vi "LVClass_HasoSlopes ctor from copy.vi"(0 "HasoSlopes in":refnum<class "HasoSlopes.lvclass">, 5 "HasoSlopes copy":refnum<class "HasoSlopes.lvclass">, 11 "error in (no error)":errorcluster) -> (4 "HasoSlopes out":refnum<class "HasoSlopes.lvclass">, 15 "error out":errorcluster)   [LabVIEW 2020, in "HasoSlopes.lvclass"]
doc: "HasoSlopes constructor from copy.\n\n--------------------------------------------------------------------------------\n\n<B>HasoSlopesIn </B> : Constant Pointer to HasoSlopes object.\n<B>HasoSlopesOut </B> : Constant Pointer to HasoSlopes object.\n<B>HasoSlopes_src </B> : Pointer to HasoSlopes object to copy.\n<B>ErrorIn </B> : Error\n<B>ErrorOut </B> : Error\n\n--------------------------------------------------------------------------------"
uses:
  HasoSlopes.lvclass
  Handle creation.ctl
  HasoSlopes.lvclass/HasoSlopes.ctl
  LVClass_HasoSlopes Read HasoSlopes _ property.vi
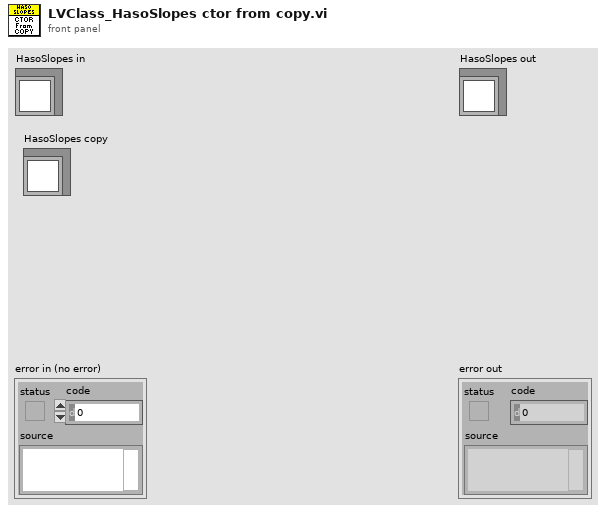
[diagram p1: front panel]
types:
  T1 = typedef "Handle creation.ctl" = enum16{"By ctor", "By write function"}
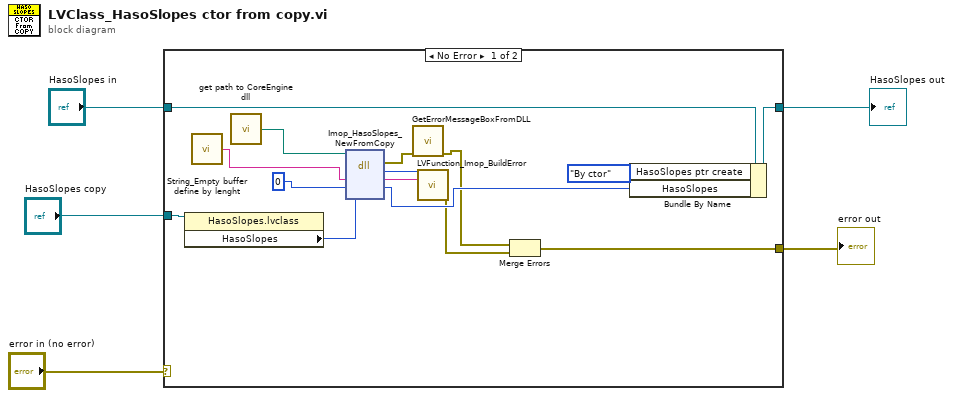
[diagram p0: block diagram]
diagram:
  n1 = case shown="No Error" "error in (no error)" {
    selector: "error in (no error)" -> [_ w22]
    tunnel: [w6 w22] -> w2
    tunnel: [w20 w21] -> w3
    tunnel: "HasoSlopes in" -> [w11 w21]
    tunnel: "HasoSlopes copy" -> [w10 _]
    frame No Error {
      n2 = property class="HasoSlopes.lvclass"(reference=w10) -> ("HasoSlopes"=w9:i32)  [unwired: 1 in, 2 out]
      n3 = call "String_Empty buffer define by lenght.vi"() -> ("Empty buffer"=w18:string)  [unwired: 1 in]
      n4 = call "get path to CoreEngine dll.vi"() -> ("path to c_interface_vc100.dll"=w19:path)  [unwired: 12 in, 3 out]
      n5 = dll-call lib="D:/soft/HASO_v3/SVN_trunk/ImOpCoreEngine4_LV2011/DLLs/c_interface_vc100.dll" fn="Imop_HasoSlopes_NewFromCopy"(path in=w19, "message"=w18, "objet"=0, "HasoSlopesCopy"=w9) -> (error out=w16:errorcluster, "return type"=w15:i32, "message"=w14:string, "objet"=w13:i32)  [unwired: 3 in, 1 out]
      n6 = call "GetErrorMessageBoxFromDLL.vi"("error IN"=w16) -> ("error OUT"=w8:errorcluster)  [unwired: 10 in]
      n7 = call "LVFunction_Imop_BuildError.vi"("code"=w15, "String to Prepend to source (\"\")"=w14) -> ("error out"=w7:errorcluster)  [unwired: 13 in]
      n8 = Merge Errors(w8, w7) -> (w6:errorcluster)
      n9 = Bundle By Name(cluster=w11, "HasoSlopes ptr create"=Handle_creation."By ctor", "HasoSlopes"=w13) -> (w20:refnum<class "HasoSlopes.lvclass">)
    }
    frame Error {
    }
  }
  "error out" <- w2
  "HasoSlopes out" <- w3
